vi "rcs.vi"(7 "RCS REF":dbl=20.9 format="%#_13g", 9 "range":dbl, 10 "rcs":dbl) -> (1 "gain":dbl, 2 "rcs result":dbl)   [LabVIEW 2015]
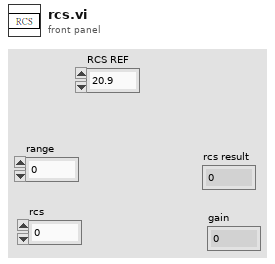
[diagram p1: front panel]
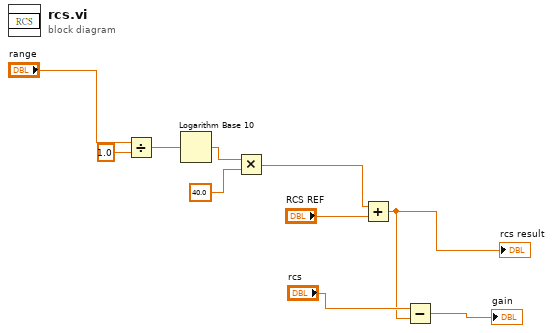
[diagram p0: block diagram]
diagram:
  n1 = Divide(x="range", y=1.0) -> (x/y=w8:dbl)
  n2 = Logarithm Base 10(1:w8) -> (0:w7:dbl)
  n3 = Multiply(x=w7, y=40.0) -> (x*y=w5:dbl)
  n4 = Add(x=w5, y="RCS REF") -> (x+y=w2:dbl)
  "rcs result" <- w2
  n5 = Subtract(x="rcs", y=w2) -> (x-y=→"gain":dbl)
